vi "cvi_get_channels.vi"(5 "arm2_channels":u8[](array[numeric]), 7 "arm1_channels":u8[](array[numeric]), 8 "error in (no error)":errorcluster, 9 "channels":u8[](array[numeric]), 10 "sync":dbl[](array[numeric]), 11 "times":dbl[](array[numeric])) -> (0 "error out":errorcluster, 2 "arm2":dbl[](array[numeric]), 3 "arm1":dbl[](array[numeric]))   [LabVIEW 2015]
uses:
  cvibuild.corr_funcs/Release/corr_funcs.dll
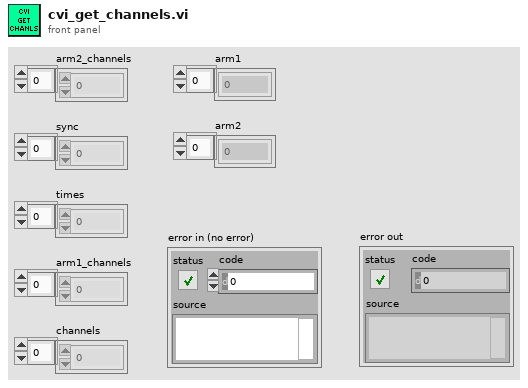
[diagram p1: front panel]
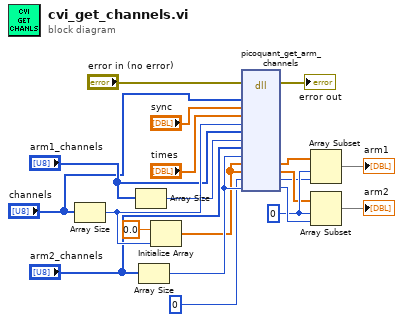
[diagram p0: block diagram]
diagram:
  w17 = 0 ("index")
  n1 = Array Size(array="channels") -> (size(s)=w10:i32)
  n2 = Array Size(array="arm1_channels") -> (size(s)=w7:i32)
  n3 = Array Size(array="arm2_channels") -> (size(s)=w13:i32)
  n4 = Initialize Array(0.0 ("element"), w10) -> (w11:dbl[])
  n5 = dll-call lib="C:/Users/bspoka/Downloads/lvoop_dll-master/cvi_project/cvibuild.corr_funcs/Release/corr_funcs.dll" fn="picoquant_get_arm_channels"(error in="error in (no error)", "channels"="channels", "sync"="sync", "times"="times", "num_records"=w10, "arm1_channels"="arm1_channels", "arm1_num"=w7, "arm2_channels"="arm2_channels", "arm2_num"=w13, "arm1"=w11, "arm2"=w11, "arm1_tally"=0, "arm2_tally"=w13) -> (error out=→"error out":errorcluster, "arm1"=w14:dbl[], "arm2"=w16:dbl[], "arm1_tally"=w15:i32, "arm2_tally"=w18:i32)  [unwired: 11 in, 1 out]
  n6 = Array Subset(array=w14, index=w17, length=w15) -> (→"arm1":dbl[])
  n7 = Array Subset(array=w16, index=w17, length=w18) -> (→"arm2":dbl[])
